vi "Configure_Compliance_ConstantSMU.vi"(7 "SMU Config":T1, 8 "error in (no error)":errorcluster, 9 "compliance (A)":dbl, 10 "compliance (V)":dbl, 11 "VISA In":refnum<visa-resource-name>) -> (0 "error out":errorcluster, 3 "VISA Out":refnum<visa-resource-name>)   [LabVIEW 2012]
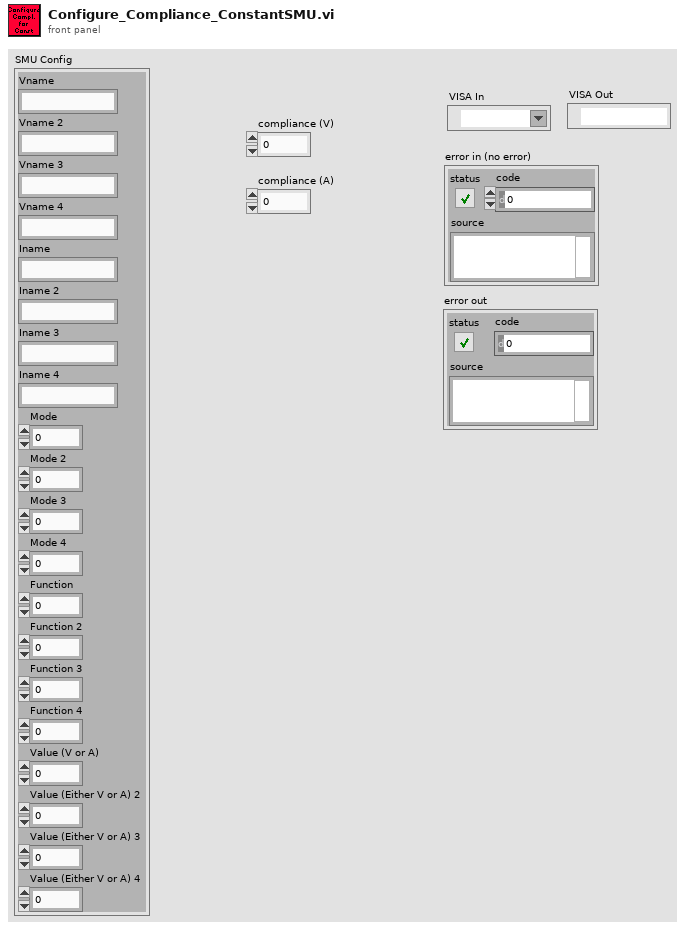
[diagram p1: front panel]
types:
  T1 = cluster{"Vname":string, "Vname 2":string, "Vname 3":string, "Vname 4":string, "Iname":string, "Iname 2":string, "Iname 3":string, "Iname 4":string, "Mode":u16, "Mode 2":u16, "Mode 3":u16, "Mode 4":u16, "Function":u16, "Function 2":u16, "Function 3":u16, "Function 4":u16, "Value (V or A)":dbl, "Value (Either V or A) 2":dbl, "Value (Either V or A) 3":dbl, "Value (Either V or A) 4":dbl}
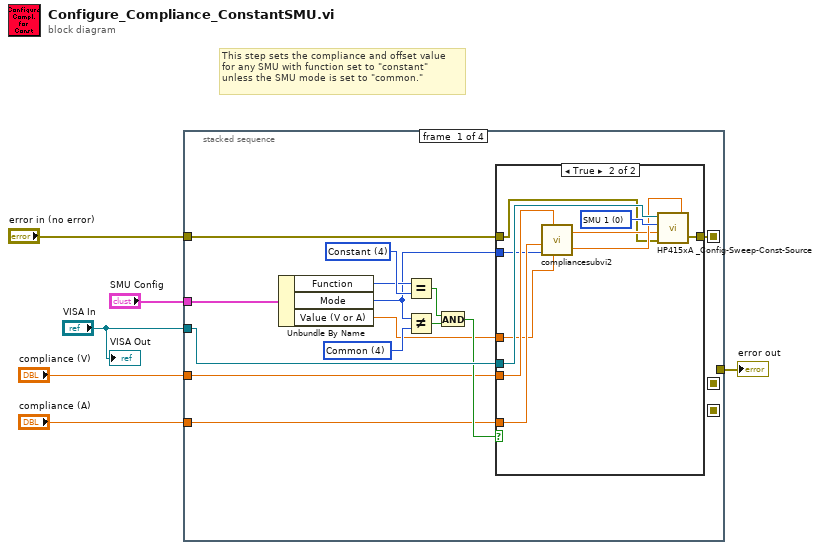
[diagram p0: block diagram]
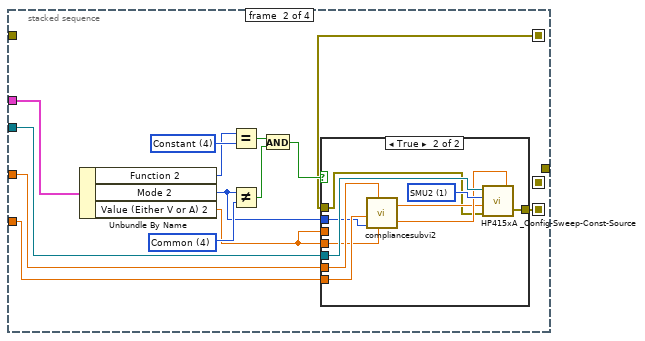
[diagram p3: hidden frame]
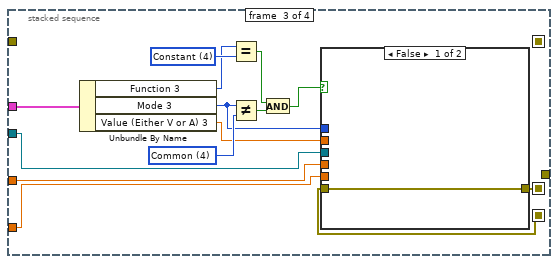
[diagram p5: hidden frame]
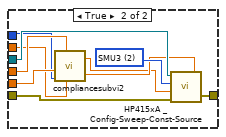
[diagram p6: hidden frame]
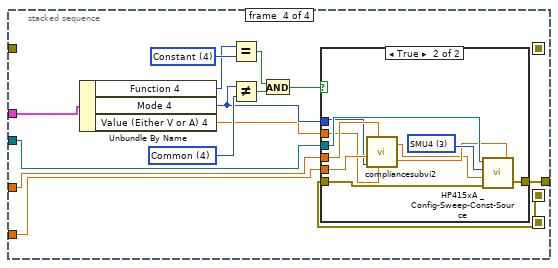
[diagram p7: hidden frame]
diagram:
  # "This step sets the compliance and offset value\nfor any SMU with function set to \"constant\"\nunless the SMU mode is set to \"common.\""
  n1 = stacked-sequence {
    seq-local: [w7 _ _ _] -> [_ w33 _ _]
    seq-local: [_ w32 _ _] -> [_ _ w58 _]
    seq-local: [_ _ w57 _] -> [_ _ _ w83]
    tunnel: "VISA In" -> [w19 w42 w66 w90]
    tunnel: "compliance (A)" -> [w14 w39 w65 w88]
    tunnel: "compliance (V)" -> [w13 w38 w64 w89]
    tunnel: "SMU Config" -> [w12 w37 w62 w87]
    tunnel: "error in (no error)" -> [w8 _ _ _]
    tunnel: [_ _ _ w82] -> w6
    frame #0 {
      w17 = u16 4 items=["V", "I", "VPulse", "IPulse", "Common"] ("Mode")
      w20 = u16 4 items=["disabled", "Var1", "Var2", "Var1'", "Constant"] ("Function")
      n2 = Unbundle By Name(w12) -> ("Function"=w10:u16, "Mode"=w9:u16, "Value (V or A)"=w11:dbl)
      n3 = Equal?(x=w10, y=w20) -> (x = y?=w18:bool)
      n4 = Not Equal?(x=w9, y=w17) -> (x != y?=w16:bool)
      n5 = And(x=w18, y=w16) -> (x .and. y?=w15:bool)
      n6 = case shown="True" w15 {
        tunnel: w19 -> [_ w31]
        tunnel: w13 -> [_ w29]
        tunnel: w14 -> [_ w28]
        tunnel: w11 -> [_ w25]
        tunnel: w9 -> [_ w26]
        tunnel: [w21 w23] -> w7
        tunnel: w8 -> [w21 w22]
        frame False {
        }
        frame True {
          w30 = u16 0 items=["SMU 1", "SMU2", "SMU3", "SMU4", "SMU5", "SMU6", "VSU1", "VSU2"] ("unit (SMU1:0)")
          n7 = call "compliancesubvi2.vi"("Value1"=w25, "compliance (V)"=w29, "Mode"=w26, "compliance (A)"=w28) -> ("compliance"=w27:dbl, "constant"=w24:dbl)  [unwired: 2 in]
          n8 = call "HP415xA _Config-Sweep-Const-Source.vi"("compliance (SMUs only)"=w27, "error in (no error)"=w22, "source (V or A)"=w24, "unit (SMU1:0)"=w30, "VISA session"=w31) -> ("error out"=w23:errorcluster)
        }
      }
    }
    frame #1 {
      w40 = u16 4 items=["V", "I", "VPulse", "IPulse", "Common"] ("Mode 2")
      w41 = u16 4 items=["disabled", "Var1", "Var2", "Var1'", "Constant"] ("Function 2")
      n9 = Unbundle By Name(w37) -> ("Function 2"=w36:u16, "Mode 2"=w35:u16, "Value (Either V or A) 2"=w34:dbl)
      n10 = Equal?(x=w36, y=w41) -> (x = y?=w45:bool)
      n11 = Not Equal?(x=w35, y=w40) -> (x != y?=w44:bool)
      n12 = And(x=w45, y=w44) -> (x .and. y?=w43:bool)
      n13 = case shown="True" w43 {
        tunnel: w42 -> [_ w56]
        tunnel: w38 -> [_ w54]
        tunnel: w39 -> [_ w53]
        tunnel: w34 -> [_ _]
        tunnel: w35 -> [_ w51]
        tunnel: w34 -> [_ w50]
        tunnel: w33 -> [w46 w48]
        tunnel: [w46 w47] -> w32
        frame False {
        }
        frame True {
          w55 = u16 1 items=["SMU 1", "SMU2", "SMU3", "SMU4", "SMU5", "SMU6", "VSU1", "VSU2"] ("unit (SMU1:0)")
          n14 = call "compliancesubvi2.vi"("Value1"=w50, "compliance (V)"=w54, "Mode"=w51, "compliance (A)"=w53) -> ("compliance"=w52:dbl, "constant"=w49:dbl)  [unwired: 2 in]
          n15 = call "HP415xA _Config-Sweep-Const-Source.vi"("compliance (SMUs only)"=w52, "error in (no error)"=w48, "source (V or A)"=w49, "unit (SMU1:0)"=w55, "VISA session"=w56) -> ("error out"=w47:errorcluster)
        }
      }
    }
    frame #2 {
      w67 = u16 4 items=["V", "I", "VPulse", "IPulse", "Common"] ("Mode 2")
      w68 = u16 4 items=["disabled", "Var1", "Var2", "Var1'", "Constant"] ("Function 2")
      n16 = Unbundle By Name(w62) -> ("Function 3"=w60:u16, "Mode 3"=w61:u16, "Value (Either V or A) 3"=w59:dbl)
      n17 = Equal?(x=w60, y=w68) -> (x = y?=w70:bool)
      n18 = Not Equal?(x=w61, y=w67) -> (x != y?=w69:bool)
      n19 = And(x=w70, y=w69) -> (x .and. y?=w63:bool)
      n20 = case shown="False" w63 {
        tunnel: w66 -> [_ w81]
        tunnel: w59 -> [_ w75]
        tunnel: w65 -> [_ w78]
        tunnel: w64 -> [_ w77]
        tunnel: w61 -> [_ w76]
        tunnel: w58 -> [w71 w73]
        tunnel: [w71 w72] -> w57
        frame False {
        }
        frame True {
          w80 = u16 2 items=["SMU 1", "SMU2", "SMU3", "SMU4", "SMU5", "SMU6", "VSU1", "VSU2"] ("unit (SMU1:0)")
          n21 = call "compliancesubvi2.vi"("Value1"=w75, "compliance (V)"=w77, "Mode"=w76, "compliance (A)"=w78) -> ("compliance"=w79:dbl, "constant"=w74:dbl)  [unwired: 2 in]
          n22 = call "HP415xA _Config-Sweep-Const-Source.vi"("compliance (SMUs only)"=w79, "error in (no error)"=w73, "source (V or A)"=w74, "unit (SMU1:0)"=w80, "VISA session"=w81) -> ("error out"=w72:errorcluster)
        }
      }
    }
    frame #3 {
      w92 = u16 4 items=["V", "I", "VPulse", "IPulse", "Common"] ("Mode 4")
      w93 = u16 4 items=["disabled", "Var1", "Var2", "Var1'", "Constant"] ("Function 4")
      n23 = Unbundle By Name(w87) -> ("Function 4"=w86:u16, "Mode 4"=w85:u16, "Value (Either V or A) 4"=w84:dbl)
      n24 = Equal?(x=w86, y=w93) -> (x = y?=w95:bool)
      n25 = Not Equal?(x=w85, y=w92) -> (x != y?=w94:bool)
      n26 = And(x=w95, y=w94) -> (x .and. y?=w91:bool)
      n27 = case shown="True" w91 {
        tunnel: w90 -> [_ w105]
        tunnel: w89 -> [_ w103]
        tunnel: w88 -> [_ w104]
        tunnel: w85 -> [_ w102]
        tunnel: w84 -> [_ w101]
        tunnel: w83 -> [w96 w98]
        tunnel: [w96 w97] -> w82
        frame False {
        }
        frame True {
          w106 = u16 3 items=["SMU 1", "SMU2", "SMU3", "SMU4", "SMU5", "SMU6", "VSU1", "VSU2"] ("unit (SMU1:0)")
          n28 = call "compliancesubvi2.vi"("Value1"=w101, "compliance (V)"=w103, "Mode"=w102, "compliance (A)"=w104) -> ("compliance"=w100:dbl, "constant"=w99:dbl)  [unwired: 2 in]
          n29 = call "HP415xA _Config-Sweep-Const-Source.vi"("compliance (SMUs only)"=w100, "error in (no error)"=w98, "source (V or A)"=w99, "unit (SMU1:0)"=w106, "VISA session"=w105) -> ("error out"=w97:errorcluster)
        }
      }
    }
  }
  "error out" <- w6
  "VISA Out" <- "VISA In"
